vi "LoadImage.vi"(1 "ImageFile":path, 5 "error in (no error)":errorcluster) -> (15 "ImageOut":refnum<k24>, 17 "ImageSize":cluster{"Width":i32, "Height":i32}, 19 "error out":errorcluster)   [LabVIEW 2020, in "LcPictureBox.lvclass"]
uses:
  <userlib>/_LabVIEWCommon/LcPictureBox_class/LcPictureBox.lvclass
  System.Drawing
  <userlib>/_LabVIEWCommon/LcPictureBox_class/LcPictureBox.lvclass/LcPictureBox.ctl
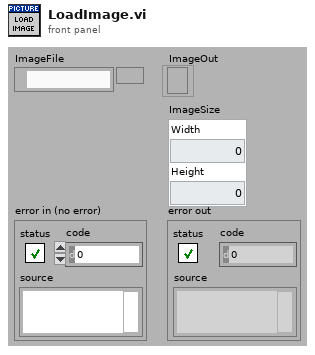
[diagram p1: front panel]
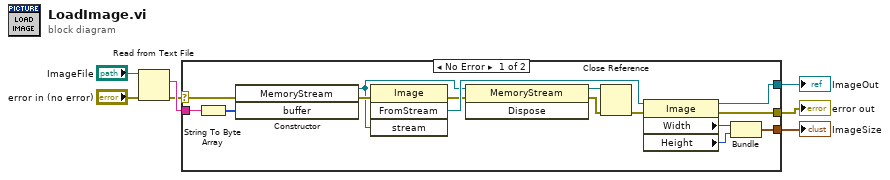
[diagram p0: block diagram]
diagram:
  n1 = Read from Text File(file (use dialog)="ImageFile", error in="error in (no error)") -> (text=w3:string, error out=w1:errorcluster)  [unwired: 2 in, 2 out]
  n2 = case shown="No Error" w1 {
    selector: w1 -> [w22 w23]
    tunnel: [w20 w23] -> w7
    tunnel: [w21 _] -> w6
    tunnel: [w17 _] -> w5
    tunnel: w3 -> [w8 _]
    frame No Error {
      n3 = String To Byte Array(string=w8) -> (unsigned byte array=w14:u8[])
      n4 = constructor class="MemoryStream"(error in=w22, "buffer"=w14) -> (reference out=w9:refnum<k24>, error out=w13:errorcluster)  [unwired: 2 in, 2 out]
      n5 = invoke class="Image" method="FromStream"(error in=w13, "stream"=w9) -> (error out=w10:errorcluster, "FromStream"=w16:refnum<k24>)  [unwired: 2 in, 2 out]
      n6 = invoke class="MemoryStream" method="Dispose"(reference=w9, error in=w10) -> (reference out=w11:refnum<k24>, error out=w12:errorcluster)  [unwired: 1 in, 1 out]
      n7 = Close Reference(reference=w11, error in (no error)=w12) -> (error out=w15:errorcluster)
      n8 = property class="Image"(reference=w16, error in=w15) -> (reference out=w21:refnum<k24>, error out=w20:errorcluster, "Width"=w19:i32, "Height"=w18:i32)
      n9 = Bundle("Width"=w19, "Height"=w18) -> (w17:cluster{"Width":i32, "Height":i32})  [unwired: 1 in]
    }
    frame Error {
    }
  }
  "error out" <- w7
  "ImageOut" <- w6
  "ImageSize" <- w5
